vi "ChargeSensingImagingGateSweep.vi"() -> ()   [LabVIEW 2021]
uses:
  <userlib>/Nanonis Prog Interface V5/Nanonis Prog Interface.lvlib
panel:
  in  "Method":u16(ring) items=["Gaussian fit", "Derivative"]
  in  "Gate increment (V)":dbl
  in  "End gate (V)":dbl
  in  "Start gate (V)":dbl
  # "KPN: Correct Imaging vs. Gate voltage program, 8/9/22"
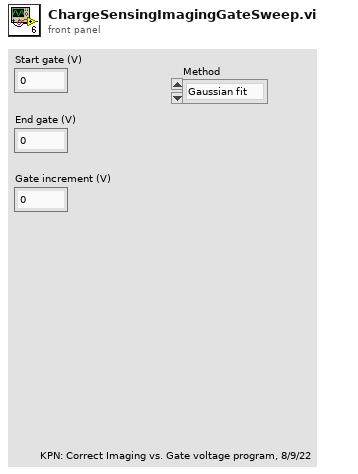
[diagram p1: front panel]
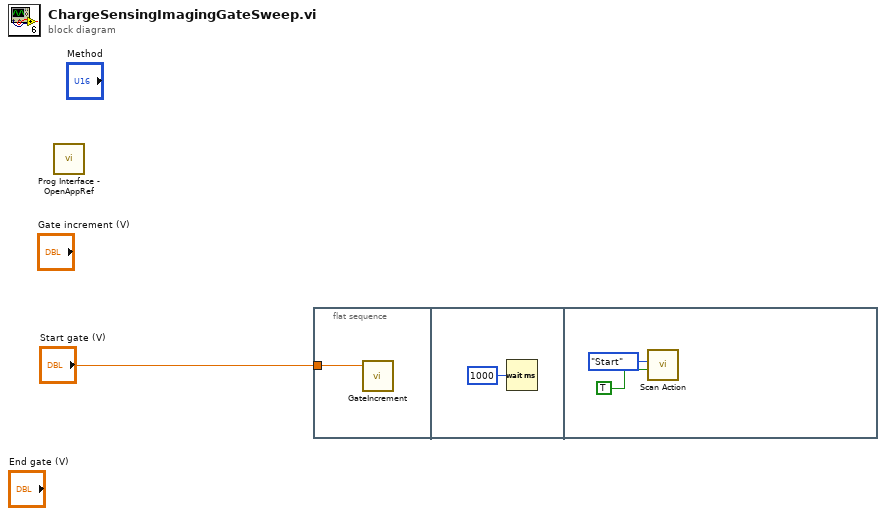
[diagram p0: block diagram]
diagram:
  n1 = call <userlib>:"Prog Interface - OpenAppRef.vi"() -> ()  [unwired: 6 in, 2 out]
  n2 = flat-sequence {
    tunnel: "Start gate (V)" -> [w2]
    frame #0 {
      n3 = call "GateIncrement.vi"("Gate Voltage"=w2) -> ()  [unwired: 11 in]
    }
    frame #1 {
      n4 = Wait (ms)(milliseconds to wait=u32 1000) -> ()  [unwired: 1 out]
    }
    frame #2 {
      n5 = call <userlib>:"Scan Action.vi"("Direction: up/down (T=up)"=TRUE, "Scan action (Start)"=enum16{"Start", "Stop", "Pause", "Resume"}."Start") -> ()  [unwired: 7 in, 2 out]
    }
  }
